vi "ChangeWhileMeasuring.vi"(5 "StopOrRestart":enum16{"StopIfMeasuring", "RestartIfMeasuring"}(ring), 6 "WasMeasuring":bool, 7 "Queue Array In":refnum<queue>[](array[refnum]), 8 "error in (no error)":errorcluster, 11 "PacificPowerSource in":refnum<class "PacificPowerSource.lvclass">) -> (0 "error out":errorcluster, 3 "PacificPowerSource out":refnum<class "PacificPowerSource.lvclass">, 4 "WasMeasuring?":bool)   [LabVIEW 2018, in "AcPwrPlugins.lvlib" / "PacificPowerSource.lvclass"]
doc: "This VI checks if the instrument is capable of send new instrument setting while the instruments is currently acquiring measurements."
uses:
  PacificPowerSource.lvclass
  Common/clMessage.ctl
  AcPwrBaseClass/AcPwrBase.lvclass
  Common/QueueTypeEnum.ctl
  Common/DequeueEnum.ctl
  Common/EnqueueEnum.ctl
  <vilib>/Utility/error.llb/Error Cluster From Error Code.vi
  <vilib>/ErrorRing/Error Ring.xnode
  AcPwrPlugins.lvlib
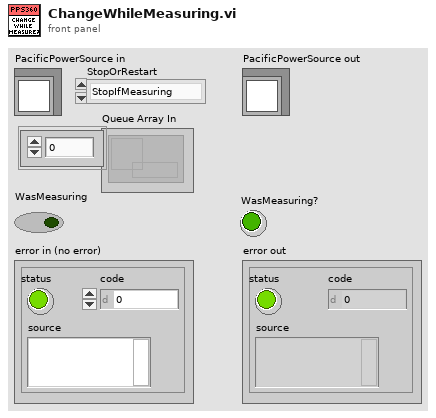
[diagram p1: front panel]
types:
  T1 = typedef "AcPwrPlugins.lvlib/DequeueEnum.ctl" = enum16{"PreviewQueue", "Dequeue"}
  T2 = typedef "AcPwrPlugins.lvlib/QueueTypeEnum.ctl" = enum16{"QMH", "Class ", "MA"}
  T3 = typedef "AcPwrPlugins.lvlib/EnqueueEnum.ctl" = enum16{"LossyEnqueue", "EnqueueAtFront", "Enqueue"}
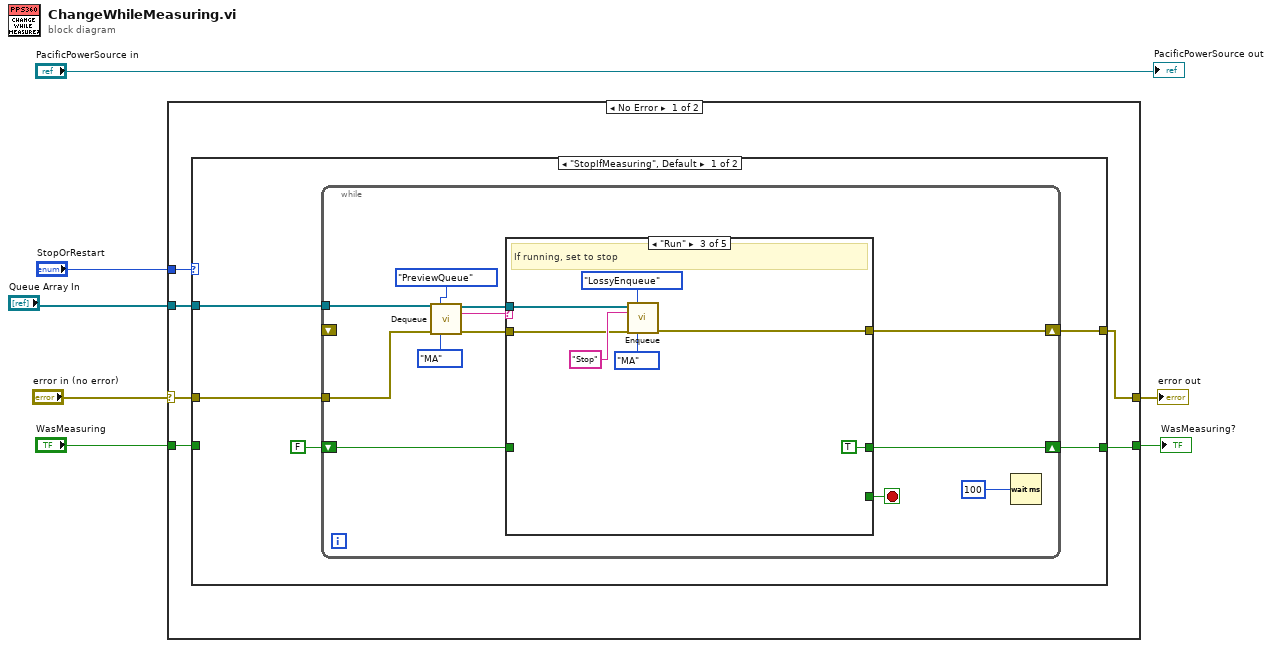
[diagram p0: block diagram]
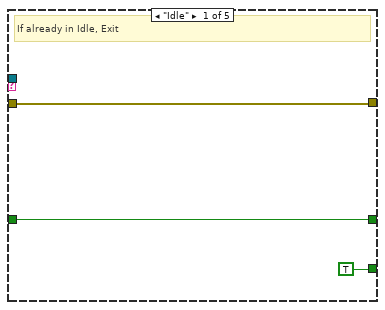
[diagram p2: hidden frame]
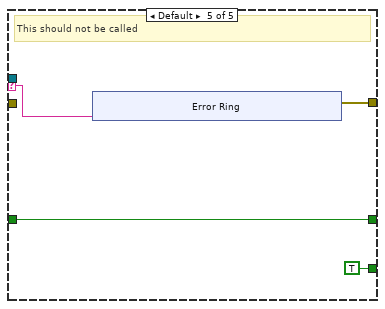
[diagram p5: hidden frame]
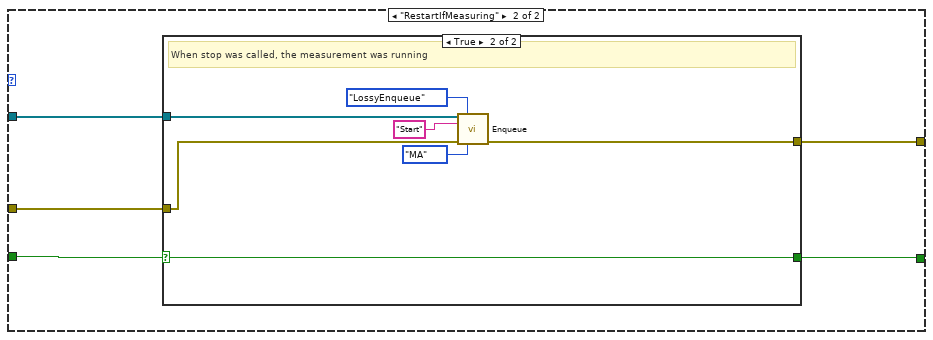
[diagram p6: hidden frame]
diagram:
  n1 = case shown="No Error" "error in (no error)" {
    selector: "error in (no error)" -> [w11 w71]
    tunnel: [w8 w71] -> w6
    tunnel: "StopOrRestart" -> [w13 _]
    tunnel: "Queue Array In" -> [w12 _]
    tunnel: "WasMeasuring" -> [w10 w70]
    tunnel: [w9 w70] -> w2
    frame No Error {
      n2 = case shown="\"StopIfMeasuring\", Default" w13 {
        tunnel: w12 -> [w15 w60]
        tunnel: w11 -> [w14 w58]
        tunnel: w10 -> [_ w59]
        tunnel: [w17 w56] -> w9
        tunnel: [w16 w57] -> w8
        frame "StopIfMeasuring", Default {
          n3 = while {
            shift-right: [w28] -> w17
            shift-left: FALSE -> [w29]
            shift-right: [w27] -> w16
            shift-left: _ -> [_]
            tunnel: w15 -> [w25]
            tunnel: w14 -> [w23]
            stop <- w26 stop-if-true
            n4 = call "Dequeue.vi"("Queue Array In"=w25, "DequeueType (PreviewQueue)"=DequeueEnum."PreviewQueue", "error in (no error)"=w23, "EnqueueType (QMH)"=QueueTypeEnum."MA") -> ("Queue Array Out"=w21:refnum<queue>[], "Message"=w20:string, "error out"=w19:errorcluster)  [unwired: 7 in, 2 out]
            n5 = case shown="\"Run\"" w20 {
              selector: w20 -> [_ _ _ _ w48]
              tunnel: w29 -> [w33 w35 _ w43 w46]
              tunnel: [w33 w35 TRUE w43 w46] -> w28
              tunnel: w21 -> [_ _ w42 _ _]
              tunnel: w19 -> [w32 w34 w38 w44 _]
              tunnel: [w32 w34 w36 w44 w47] -> w27
              tunnel: [TRUE _ _ _ TRUE] -> w26
              frame "Idle" {
                # "If already in Idle, Exit"
              }
              frame "Start" {
                # "If just starting, wait 100 ms and check again"
              }
              frame "Run" {
                # "If running, set to stop"
                n6 = call "Enqueue.vi"("Queue Array In"=w42, "EnqueueType (Enqueue)"=EnqueueEnum."LossyEnqueue", "Message"="Stop", "error in (no error)"=w38, "EnqueueType (QMH)"=QueueTypeEnum."MA") -> ("error out"=w36:errorcluster)  [unwired: 8 in, 2 out]
              }
              frame "Stop" {
                # "If stopping, wait 100 ms and check again"
              }
              frame Default {
                # "This should not be called"
                n7 = xnode "Error Ring"("parameter 0"=w48) -> ("error out"=w47:errorcluster)
              }
            }
            n8 = Wait (ms)(milliseconds to wait=u32 100) -> ()  [unwired: 1 out]
          }
        }
        frame "RestartIfMeasuring" {
          n9 = case shown="True" w59 {
            selector: w59 -> [w61 w63]
            tunnel: w60 -> [_ w66]
            tunnel: w58 -> [w62 w65]
            tunnel: [w62 w64] -> w57
            tunnel: [w61 w63] -> w56
            frame False {
              # "When stop was called, the Measurement was in Idle"
            }
            frame True {
              # "When stop was called, the measurement was running"
              n10 = call "Enqueue.vi"("Queue Array In"=w66, "EnqueueType (Enqueue)"=EnqueueEnum."LossyEnqueue", "Message"="Start", "error in (no error)"=w65, "EnqueueType (QMH)"=QueueTypeEnum."MA") -> ("error out"=w64:errorcluster)  [unwired: 8 in, 2 out]
            }
          }
        }
      }
    }
    frame Error {
    }
  }
  "error out" <- w6
  "WasMeasuring?" <- w2
  "PacificPowerSource out" <- "PacificPowerSource in"
